vi "createDAQ.vi"(0 "device":string="Dev1") -> (7 "function return":u32)   [LabVIEW 2020]
uses:
  cDaqlib/cDaq.lvlib
panel:
  in  "digital_co_io_id":i32[](array[numeric])=array[4097 elements]
  in  "analog_co_count":i32=1
  in  "digital_io_id":i32[](array[numeric])=array[4097 elements]
  in  "analog_co_io_id":i32[](array[numeric])=array[4097 elements]
  in  "digital_count":i32=1
  in  "analog_io_id":i32[](array[numeric])=array[4097 elements]
  in  "analog_count":i32=1
  in  "digital_co_count":i32
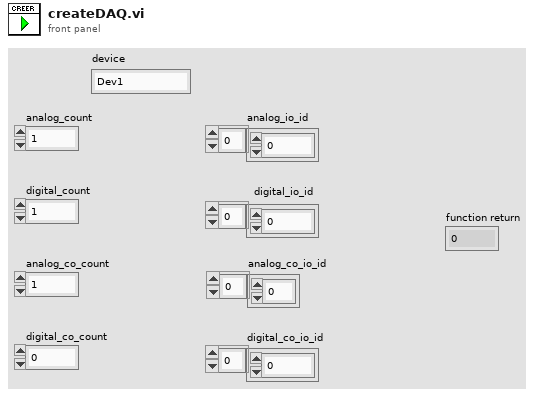
[diagram p1: front panel]
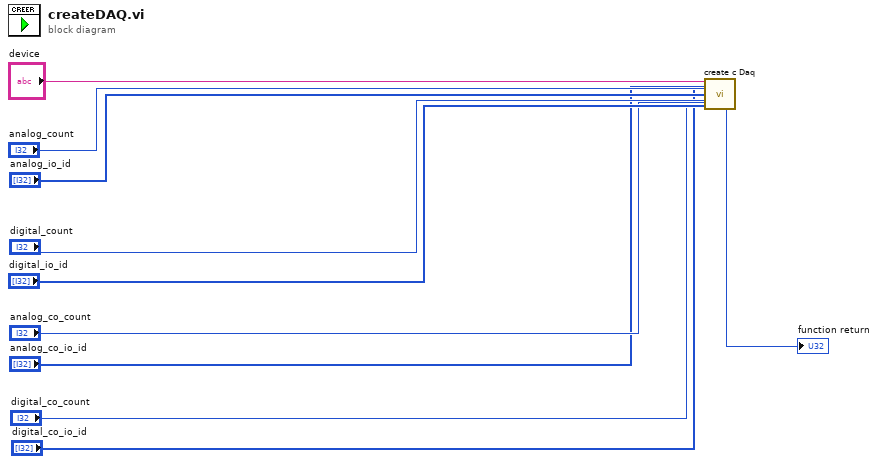
[diagram p0: block diagram]
diagram:
  n1 = call "create c Daq.vi"("device"="device", "digital_io_id"="digital_io_id", "analog_co_io_id"="analog_co_io_id", "digital_co_io_id"="digital_co_io_id", "analog_count"="analog_count", "analog_io_id"="analog_io_id", "digital_count"="digital_count", "analog_co_count"="analog_co_count", "digital_co_count"="digital_co_count") -> ("function return"=→"function return":u32)  [unwired: 2 in, 4 out]
